vi "tsflexray_start_net.vi"(8 "error in (no error)":errorcluster caption="错误输入（无错误）", 9 "ATimeoutMs":i32, 10 "AIdxChn":i32, 11 "路径输入":path) -> (0 "error out":errorcluster caption="错误输出", 2 "function return":i32, 3 "路径输出":path)   [LabVIEW 2014]
doc: "TSAPI(s32)tsflexray_start_net(const s32 AIdxChn,const s32 ATimeoutMs);"
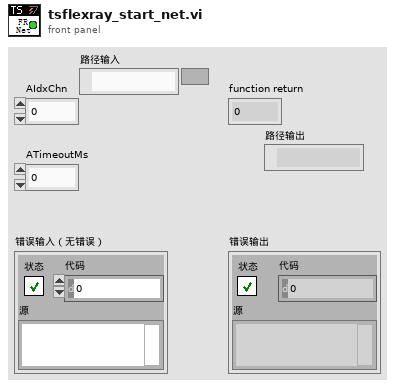
[diagram p1: front panel]
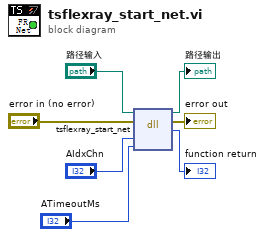
[diagram p0: block diagram]
diagram:
  n1 = dll-call lib="D:/Work/LabVIEW Code/TSMaster Labview SDK/LabVIEW/LabVIEW-TSMasterAPI_CLN/TSMasterAPI_LabVIEW-2024-10-08 14-20-13/Not_organized_vi/TSMaster.*" fn="tsflexray_start_net"(path in="路径输入", error in="error in (no error)", "AIdxChn"="AIdxChn", "ATimeoutMs"="ATimeoutMs") -> (path out=→"路径输出":path, error out=→"error out":errorcluster, "返回类型"=→"function return":i32)  [unwired: 3 in]
